vi "error.vi"(0 "result code":i32, 5 "error in (no error)":errorcluster, 7 "ignore range violation":bool, 9 "size trace log":u32=1000, 11 "call trace log":bool) -> (13 "trace log":string, 14 "status":string, 19 "error out":errorcluster)   [LabVIEW 2010, in "OSA.lvclass"]
doc: "SubVI to a <B>Thorlabs_OSA_64</B> object.\n\n[GOOP 1.0]"
uses:
  OSA.lvclass
  typeDef/fts_error.ctl
  OSA20X_misc.lvlib
  FTSLib.dll
panel:
  out "tracebuffer returnVal":i32
  in  "result":T1=[{"nr"=0, "error"="FTS_SUCCESS"}, {"nr"=1, "error"="FTS_ERROR_NOT_IMPLEMENTED"}, {"nr"=2, "error"="FTS_ERROR_NOT_WRITABLE"}, {"nr"=3, "error"="FTS_ERROR_RANGE_ERROR"}, {"nr"=4, "error"="FTS_ERROR_CMD_IGNORED"}, {"nr"=10, "error"="FTS_ERROR_INVALID_CONFIGURATION"}, {"nr"=64, "error"="FTS_ERROR_COMMUNICATION_FAILURE"}, {"nr"=65, "error"="FTS_ERROR_TIMEOUT"}, {"nr"=66, "error"="FTS_ERROR_SPECTROMETER_FAILURE"}, {"nr"=67, "error"="FTS_ERROR_SPECTROMETER_BUSY"}, {"nr"=68, "error"="FTS_ERROR_COMMUNICATION_NOT_OPENED"}, {"nr"=69, "error"="FTS_ERROR_SPECTROMETER_NOT_FOUND"}, {"nr"=70, "error"="FTS_ERROR_IN_SETTINGS"}, {"nr"=256, "error"="FTS_ERROR_PARAMETER_ERROR"}, {"nr"=257, "error"="FTS_ERROR_DATA_ERROR"}, {"nr"=258, "error"="FTS_ERROR_NOT_POWEROFTWO"}, {"nr"=259, "error"="FTS_ERROR_DIMENSION_MISMATCH"}, {"nr"=260, "error"="FTS_ERROR_OUTOFMEMORY"}, {"nr"=275, "error"="FTS_ERROR_SATURATED_INTERFEROGRAM"}, {"nr"=276, "error"="FTS_ERROR_INTERFEROGRAM_INTENSITY_LOW"}] {"nr" format="%x"}
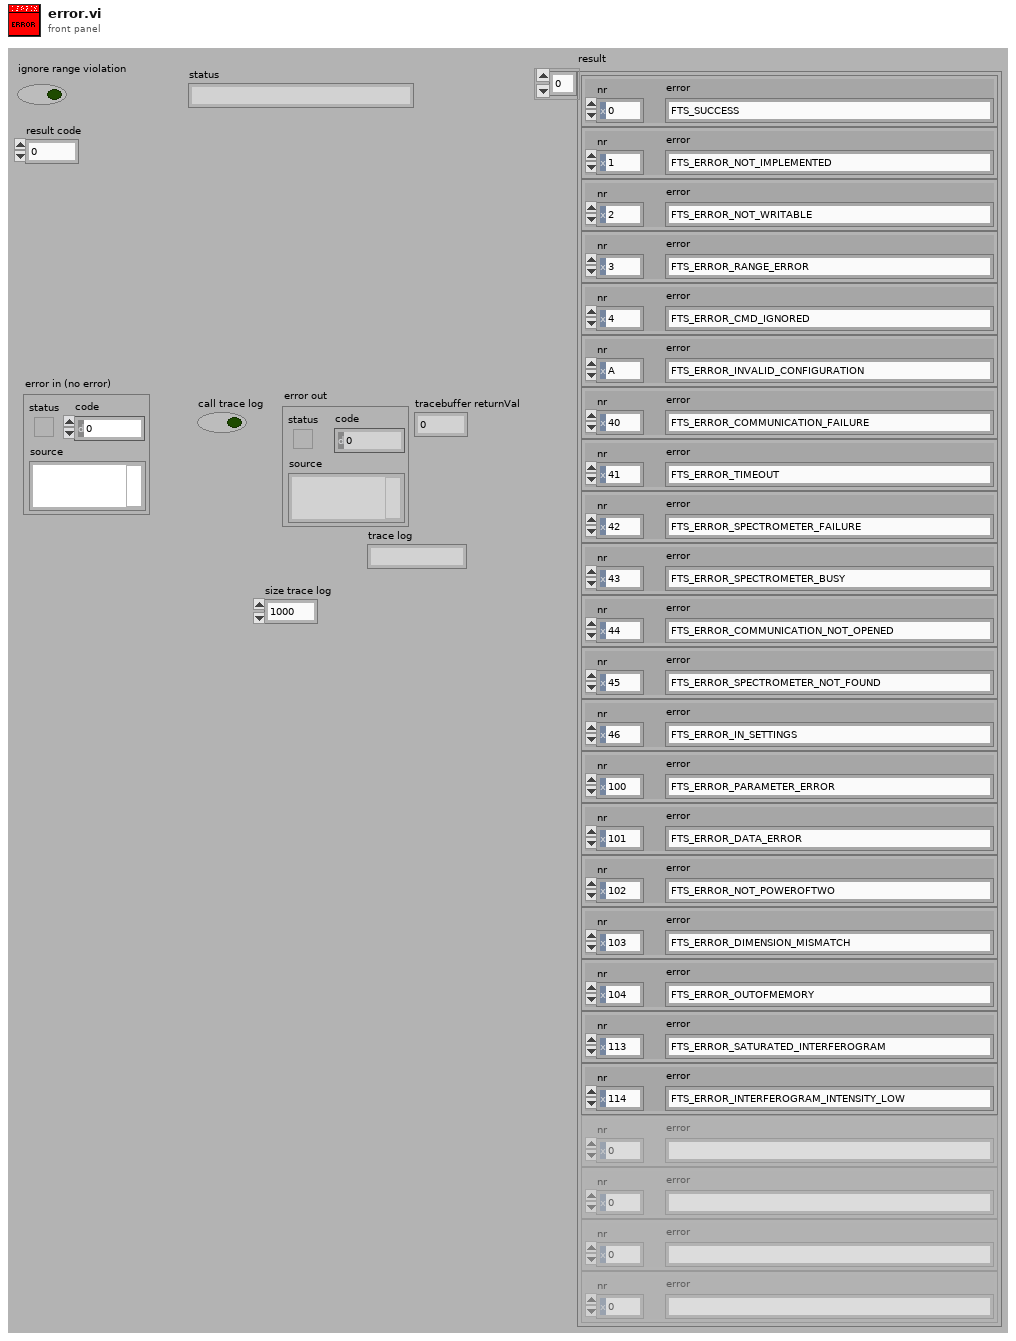
[diagram p1: front panel]
types:
  T1 = typedef "OSA.lvclass/fts_error.ctl" = cluster{"nr":i32, "error":string}[]
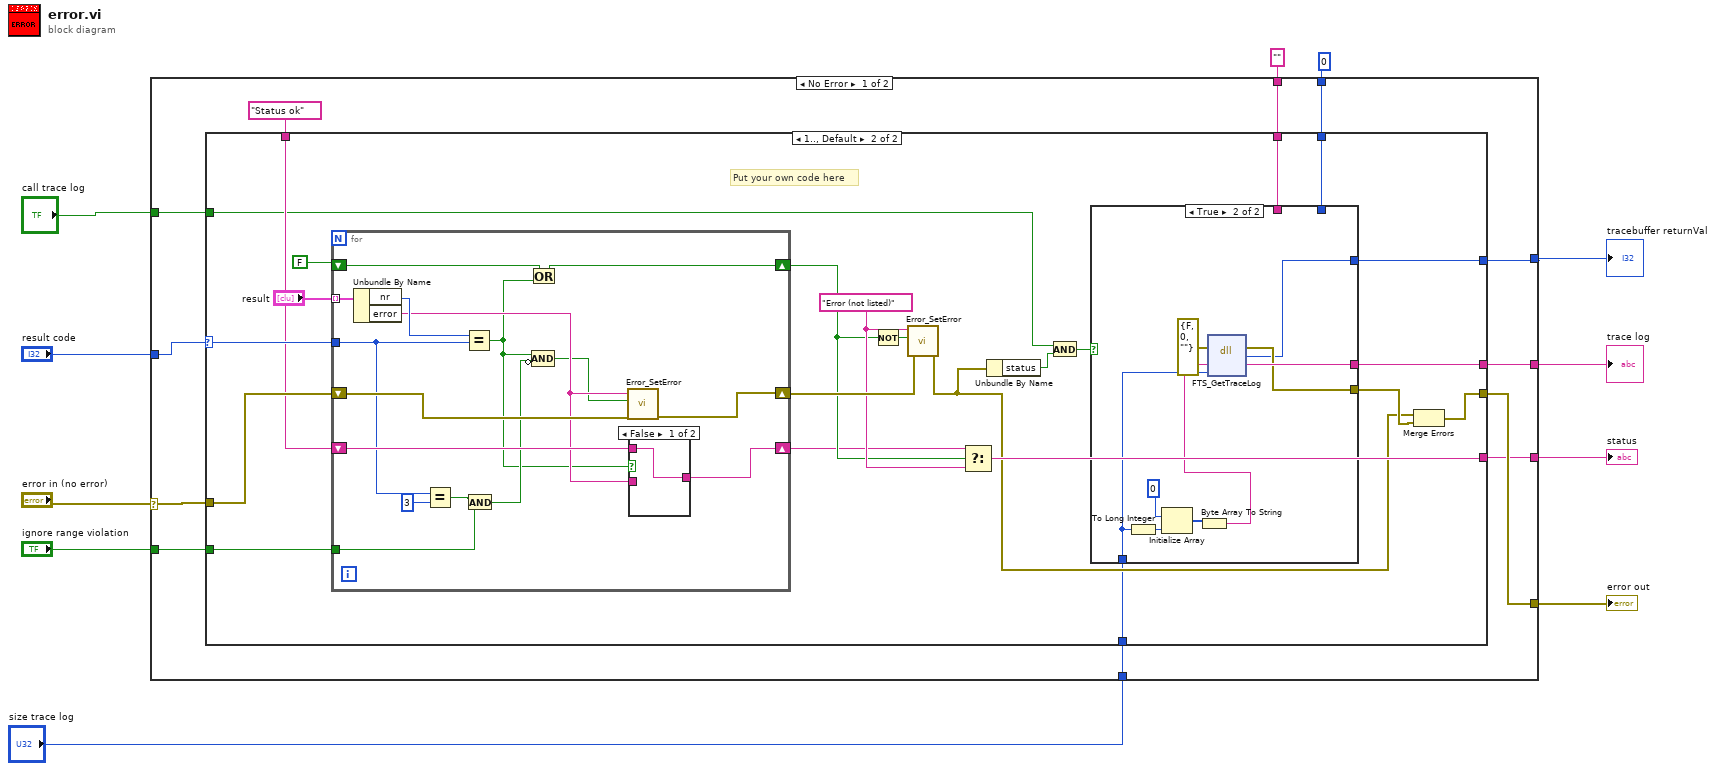
[diagram p0: block diagram]
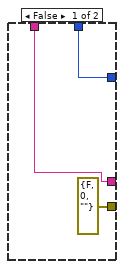
[diagram p3: hidden frame]
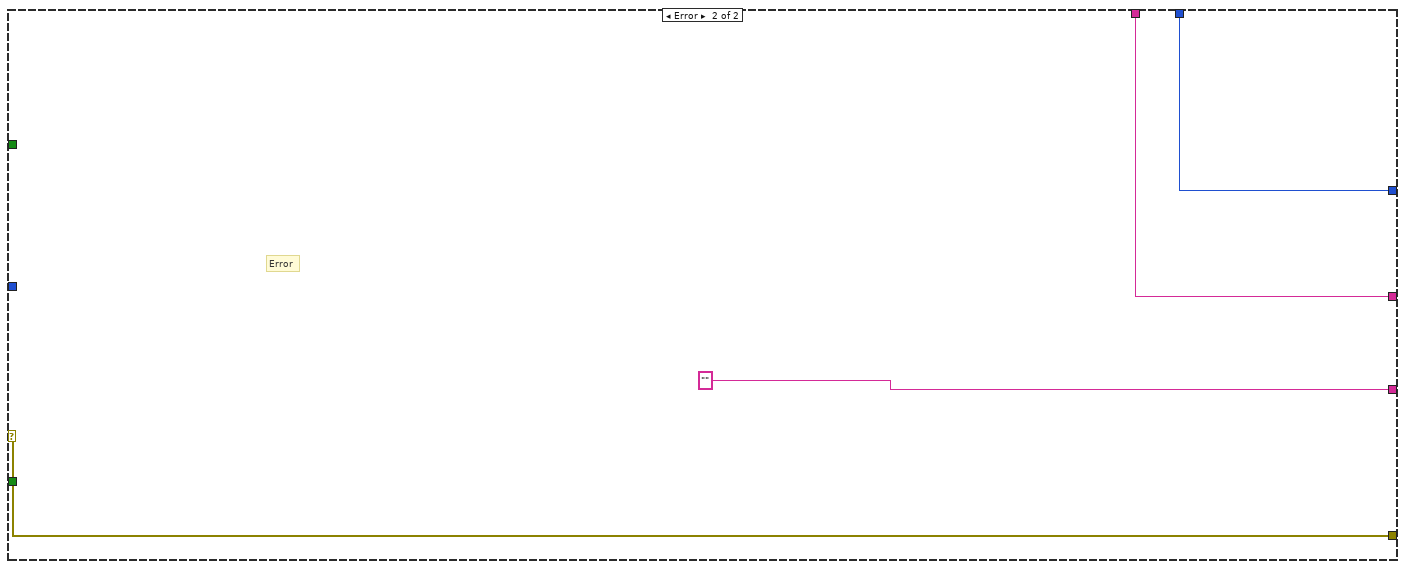
[diagram p5: hidden frame]
diagram:
  n1 = case shown="No Error" "error in (no error)" {
    selector: "error in (no error)" -> [w23 w84]
    tunnel: [w22 w84] -> w11
    tunnel: "result code" -> [w21 _]
    tunnel: [w20 ""] -> w8
    tunnel: "ignore range violation" -> [w19 _]
    tunnel: "call trace log" -> [w17 _]
    tunnel: [w16 w81] -> w5
    tunnel: [w15 w82] -> w4
    tunnel: "" ("buffer") -> [w14 w81]
    tunnel: 0 ("returnVal") -> [w13 w82]
    tunnel: "size trace log" -> [w12 _]
    frame No Error {
      n2 = case shown="1.., Default" w21 {
        selector: w21 -> [_ w49]
        tunnel: w23 -> [w27 w48]
        tunnel: [w27 w32] -> w22
        tunnel: [w26 w40] -> w20
        tunnel: w19 -> [_ w47]
        tunnel: "Status ok" -> [w26 w46]
        tunnel: w17 -> [_ w37]
        tunnel: [w25 w35] -> w16
        tunnel: [w24 w31] -> w15
        tunnel: w14 -> [w25 w30]
        tunnel: w13 -> [w24 w29]
        tunnel: w12 -> [_ w28]
        frame 0 {
        }
        frame 1.., Default {
          w43 = "Error (not listed)" ("source(\"\")")
          # "Put your own code here"
          n3 = for {
            tunnel: "result" -> [w78] mode=indexing
            tunnel: w49 -> [w70]
            shift-right: [w75] -> w44
            shift-left: w48 -> [w76]
            shift-right: [w73] -> w41
            shift-left: w46 -> [w74]
            tunnel: w47 -> [w68]
            shift-right: [w64] -> w42
            shift-left: FALSE -> [w63]
            n4 = Unbundle By Name(w78) -> ("nr"=w77:i32, "error"=w72:string)
            n5 = Equal?(x=w70, y=3) -> (x = y?=w69:bool)
            n6 = Equal?(x=w77, y=w70) -> (x = y?=w65:bool)
            n7 = And(x=w69, y=w68) -> (x .and. y?=w67:bool)
            n8 = Or(x=w63, y=w65) -> (x .or. y?=w64:bool)
            n9 = Compound Arithmetic op=AND(w65, invert w67) -> (w66:bool)
            n10 = call "Error_SetError.vi"("error in"=w76, "status (true)"=w66, "source(\"\")"=w72) -> ("error out"=w75:errorcluster)  [unwired: 4 in]
            n11 = case shown="False" w65 {
              tunnel: w74 -> [w79 _]
              tunnel: [w79 w80] -> w73
              tunnel: w72 -> [_ w80]
              frame False {
              }
              frame True {
              }
            }
          }
          n12 = Not(x=w42) -> (.not. x?=w39:bool)
          n13 = call "Error_SetError.vi"("error in"=w44, "status (true)"=w39, "source(\"\")"=w43) -> ("error out"=w33:errorcluster)  [unwired: 4 in]
          n14 = Select(t=w41, s=w42, f=w43) -> (s? t:f=w40:string)
          n15 = Unbundle By Name(w33) -> ("status"=w38:bool)
          n16 = And(x=w37, y=w38) -> (x .and. y?=w36:bool)
          n17 = case shown="True" w36 {
            tunnel: [w52 w59] -> w35
            tunnel: [errorcluster {"status"=FALSE, "code"=0, "source"=""} ("error out") w58] -> w34
            tunnel: [w51 w56] -> w31
            tunnel: w30 -> [w52 _]
            tunnel: w29 -> [w51 _]
            tunnel: w28 -> [_ w55]
            frame False {
            }
            frame True {
              n18 = To Long Integer(number=w55) -> (32bit integer=w54:i32)
              n19 = Initialize Array(u8 0, w54) -> (w61:u8[])
              n20 = Byte Array To String(unsigned byte array=w61) -> (string=w60:string)
              n21 = dll-call lib="FTSLib.dll" fn="FTS_GetTraceLog"(error in=errorcluster {"status"=FALSE, "code"=0, "source"=""} ("error in (no error)"), "buffer"=w60, "buffer_length"=w55) -> (error out=w58:errorcluster, "returnVal"=w56:i32, "buffer"=w59:string)  [unwired: 3 in, 1 out]
            }
          }
          n22 = Merge Errors(w33, w34) -> (w32:errorcluster)
        }
      }
    }
    frame Error {
      # "Error"
    }
  }
  "error out" <- w11
  "status" <- w8
  "trace log" <- w5
  "tracebuffer returnVal" <- w4
